vi "Build XML Filename.vi"(9 "Xml Filename In":string, 10 "SubFolder In":string, 11 "Folder In":string) -> (3 "Full Filename Out":path)   [LabVIEW 2024, in "LVarex.lvlib"]
uses:
  LVarex.lvlib
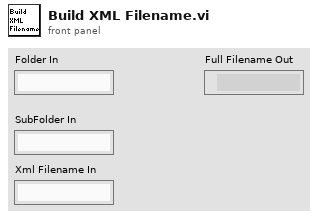
[diagram p1: front panel]
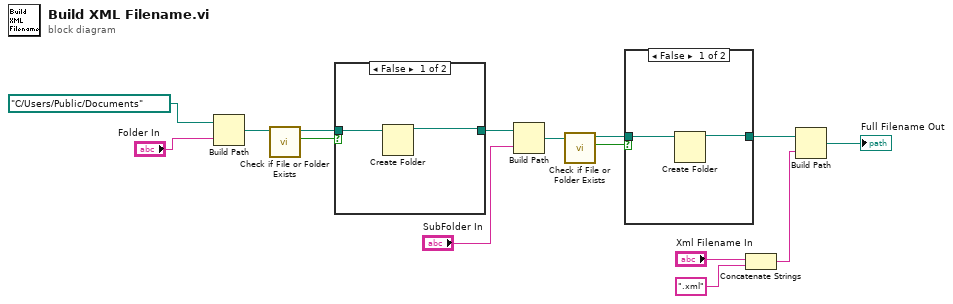
[diagram p0: block diagram]
diagram:
  n1 = Build Path(base path=path "C:/Users/Public/Documents", name or relative path="Folder In") -> (appended path=w13:path)
  n2 = call <vilib>:"Check if File or Folder Exists.vi"("path"=w13) -> ("file or folder exists?"=w12:bool, "dup path"=w11:path)  [unwired: 8 in, 1 out]
  n3 = case shown="False" w12 {
    tunnel: w11 -> [w17 w18]
    tunnel: [w16 w18] -> w10
    frame False {
      n4 = Create Folder(path (use dialog)=w17) -> (created path=w16:path)  [unwired: 2 in, 2 out]
    }
    frame True {
    }
  }
  n5 = Build Path(base path=w10, name or relative path="SubFolder In") -> (appended path=w8:path)
  n6 = call <vilib>:"Check if File or Folder Exists.vi"("path"=w8) -> ("file or folder exists?"=w7:bool, "dup path"=w6:path)  [unwired: 8 in, 1 out]
  n7 = case shown="False" w7 {
    tunnel: w6 -> [w20 w21]
    tunnel: [w19 w21] -> w5
    frame False {
      n8 = Create Folder(path (use dialog)=w20) -> (created path=w19:path)  [unwired: 2 in, 2 out]
    }
    frame True {
    }
  }
  n9 = Concatenate Strings("Xml Filename In", ".xml") -> (w2:string)
  n10 = Build Path(base path=w5, name or relative path=w2) -> (appended path=→"Full Filename Out":path)
